vi "JSONToSample.vi"(8 "ErrorIn":errorcluster, 11 "JSONIn":refnum<class "JSON Value.lvclass">) -> (0 "ErrorOut":errorcluster, 2 "Sample":T1, 3 "JSONOut":refnum<class "JSON Value.lvclass">)   [LabVIEW 2016]
doc: "Convert JSON to Sample."
uses:
  <vilib>/addons/JSON API/JSON Value/JSON Value.lvclass
  FallSensor/Sample.ctl
  FallSensor/Reading.ctl
  <vilib>/addons/JSON API/JSON Value/Get Object Item by Name.vi
  <vilib>/addons/JSON API/JSON Scalar/Get as I32.vi
  <vilib>/addons/JSON API/Get Polymorphic/JSON GetSet.lvlib
  <vilib>/addons/JSON API/JSON Scalar/JSON Scalar.lvclass
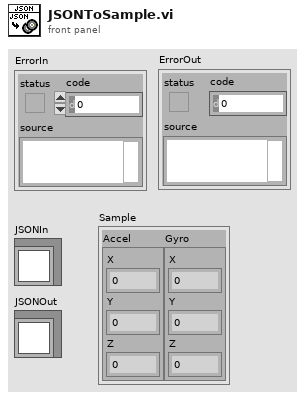
[diagram p1: front panel]
types:
  T1 = typedef "Sample.ctl" = cluster{"Accel":T2, "Gyro":T2}
  T2 = typedef "Reading.ctl" = cluster{"X":i16, "Y":i16, "Z":i16}
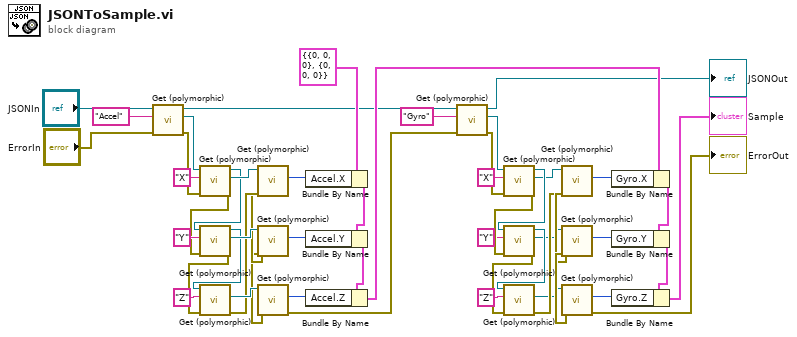
[diagram p0: block diagram]
diagram:
  n1 = call-poly <vilib>:"Get (polymorphic).vi"("error in (no error)"="ErrorIn", "name"="Accel", "JSON Value In"="JSONIn") -> ("error out"=w35:errorcluster, "Value"=w45:refnum<class "JSON Value.lvclass">, "JSON Value Out"=w5:refnum<class "JSON Value.lvclass">)  [unwired: 5 in, 1 out]
  n2 = call-poly <vilib>:"Get (polymorphic).vi"("error in (no error)"=w35, "name"="X", "JSON Value In"=w45) -> ("error out"=w34:errorcluster, "Value"=w43:refnum<class "JSON Value.lvclass">, "JSON Value Out"=w40:refnum<class "JSON Value.lvclass">)  [unwired: 5 in, 1 out]
  n3 = call-poly <vilib>:"Get (polymorphic).vi"("error in (no error)"=w34, "name"="Y", "JSON Value In"=w40) -> ("error out"=w33:errorcluster, "Value"=w39:refnum<class "JSON Value.lvclass">, "JSON Value Out"=w38:refnum<class "JSON Value.lvclass">)  [unwired: 5 in, 1 out]
  n4 = call-poly <vilib>:"Get (polymorphic).vi"("error in (no error)"=w33, "name"="Z", "JSON Value In"=w38) -> ("error out"=w32:errorcluster, "Value"=w37:refnum<class "JSON Value.lvclass">)  [unwired: 5 in, 2 out]
  n5 = call-poly <vilib>:"Get (polymorphic).vi"("error in (no error)"=w32, "JSON Scalar in"=w43) -> ("error out"=w31:errorcluster, "Number"=w50:i32)  [unwired: 7 in, 1 out]
  n6 = call-poly <vilib>:"Get (polymorphic).vi"("error in (no error)"=w31, "JSON Scalar in"=w39) -> ("error out"=w30:errorcluster, "Number"=w49:i32)  [unwired: 7 in, 1 out]
  n7 = call-poly <vilib>:"Get (polymorphic).vi"("error in (no error)"=w30, "JSON Scalar in"=w37) -> ("error out"=w3:errorcluster, "Number"=w48:i32)  [unwired: 7 in, 1 out]
  n8 = Bundle By Name(cluster=T1 {"Accel"={"X"=0, "Y"=0, "Z"=0}, "Gyro"={"X"=0, "Y"=0, "Z"=0}} ("Sample"), "Accel.X"=w50) -> (w47:T1)
  n9 = Bundle By Name(cluster=w47, "Accel.Y"=w49) -> (w46:T1)
  n10 = Bundle By Name(cluster=w46, "Accel.Z"=w48) -> (w8:T1)
  n11 = call-poly <vilib>:"Get (polymorphic).vi"("error in (no error)"=w3, "name"="Gyro", "JSON Value In"=w5) -> ("error out"=w24:errorcluster, "Value"=w15:refnum<class "JSON Value.lvclass">, "JSON Value Out"=→"JSONOut":refnum<class "JSON Value.lvclass">)  [unwired: 5 in, 1 out]
  n12 = call-poly <vilib>:"Get (polymorphic).vi"("error in (no error)"=w24, "name"="X", "JSON Value In"=w15) -> ("error out"=w25:errorcluster, "Value"=w17:refnum<class "JSON Value.lvclass">, "JSON Value Out"=w20:refnum<class "JSON Value.lvclass">)  [unwired: 5 in, 1 out]
  n13 = call-poly <vilib>:"Get (polymorphic).vi"("error in (no error)"=w25, "name"="Y", "JSON Value In"=w20) -> ("error out"=w26:errorcluster, "Value"=w21:refnum<class "JSON Value.lvclass">, "JSON Value Out"=w22:refnum<class "JSON Value.lvclass">)  [unwired: 5 in, 1 out]
  n14 = call-poly <vilib>:"Get (polymorphic).vi"("error in (no error)"=w26, "name"="Z", "JSON Value In"=w22) -> ("error out"=w27:errorcluster, "Value"=w23:refnum<class "JSON Value.lvclass">)  [unwired: 5 in, 2 out]
  n15 = call-poly <vilib>:"Get (polymorphic).vi"("error in (no error)"=w27, "JSON Scalar in"=w17) -> ("error out"=w28:errorcluster, "Number"=w10:i32)  [unwired: 7 in, 1 out]
  n16 = call-poly <vilib>:"Get (polymorphic).vi"("error in (no error)"=w28, "JSON Scalar in"=w21) -> ("error out"=w29:errorcluster, "Number"=w11:i32)  [unwired: 7 in, 1 out]
  n17 = call-poly <vilib>:"Get (polymorphic).vi"("error in (no error)"=w29, "JSON Scalar in"=w23) -> ("error out"=→"ErrorOut":errorcluster, "Number"=w12:i32)  [unwired: 7 in, 1 out]
  n18 = Bundle By Name(cluster=w8, "Gyro.X"=w10) -> (w13:T1)
  n19 = Bundle By Name(cluster=w13, "Gyro.Y"=w11) -> (w14:T1)
  n20 = Bundle By Name(cluster=w14, "Gyro.Z"=w12) -> (→"Sample":T1)
